vi "题目3.vi"(2 "温度单位":bool, 3 "停止":bool) -> (0 "温度计":dbl(slide) scale=0.0..100.0, 1 "字符串":string)   [LabVIEW 2017]
panel:
  # "°F"
  # "°C"
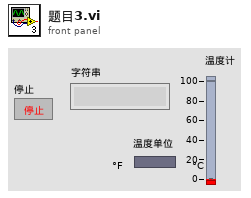
[diagram p1: front panel]
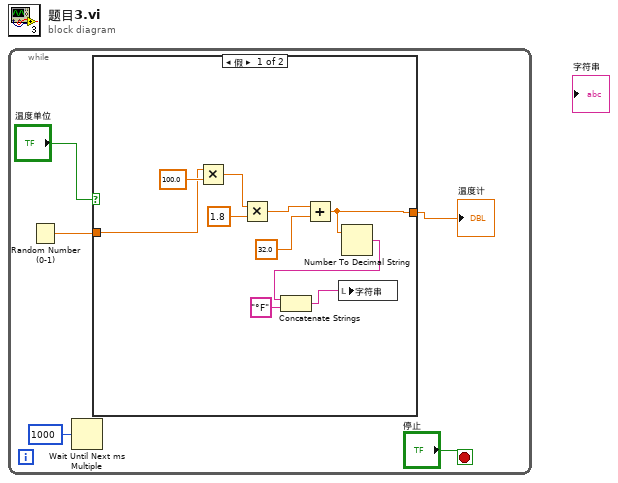
[diagram p0: block diagram]
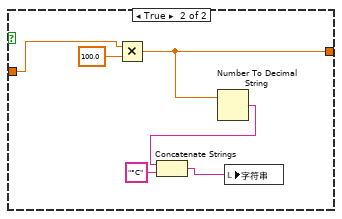
[diagram p2: hidden frame]
diagram:
  n1 = while {
    stop <- "停止" stop-if-true
    n2 = Random Number (0-1)() -> (number: 0 to 1=w3:dbl)
    n3 = Wait Until Next ms Multiple(millisecond multiple=u32 1000 ("毫秒倍数")) -> ()  [unwired: 1 out]
    n4 = case shown="假" "温度单位" {
      tunnel: [w8 w16] -> w1
      tunnel: w3 -> [w10 w20]
      frame False {
        n5 = Multiply(x=w10, y=100.0) -> (x*y=w11:dbl)
        n6 = Multiply(x=w11, y=1.8) -> (x*y=w13:dbl)
        n7 = Add(x=w13, y=32.0) -> (x+y=w8:dbl)
        n8 = Number To Decimal String(number=w8) -> (decimal integer string=w7:string)  [unwired: 1 in]
        n9 = Concatenate Strings(w7, "°F" ("字符串")) -> (w9:string)
        n10 = local write "字符串"(w9) -> ()
      }
      frame True {
        n11 = Multiply(x=w20, y=100.0) -> (x*y=w16:dbl)
        n12 = Number To Decimal String(number=w16) -> (decimal integer string=w19:string)  [unwired: 1 in]
        n13 = Concatenate Strings(w19, "°C" ("字符串")) -> (w17:string)
        n14 = local write "字符串"(w17) -> ()
      }
    }
    "温度计" <- w1
  }
